vi "LHF.DB.Mongo.Util.BSONEnumToVariantArray.vi"(0 "BsonENUM":refnum<k24>, 1 "Extract _id":bool, 5 "error in (no error)":errorcluster, 8 "type":variant) -> (14 "Documents":variant[](array[variant]), 15 "ObjectIDs":string[](array[string]), 19 "error out":errorcluster)   [LabVIEW 2013, in "LHF.DB.Mongo.lvclass"]
uses:
  LHF.DB.Mongo.lvclass
  C:/Users/Ricardo/Desktop/Projetos/LabVIEW-MongoDB/src/Driver/MongoDB.Bson.dll
  Driver/MongoDB.Bson.dll
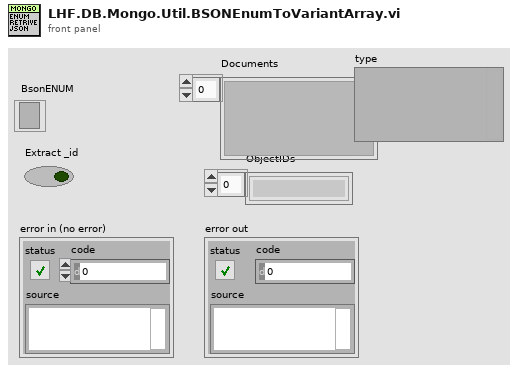
[diagram p1: front panel]
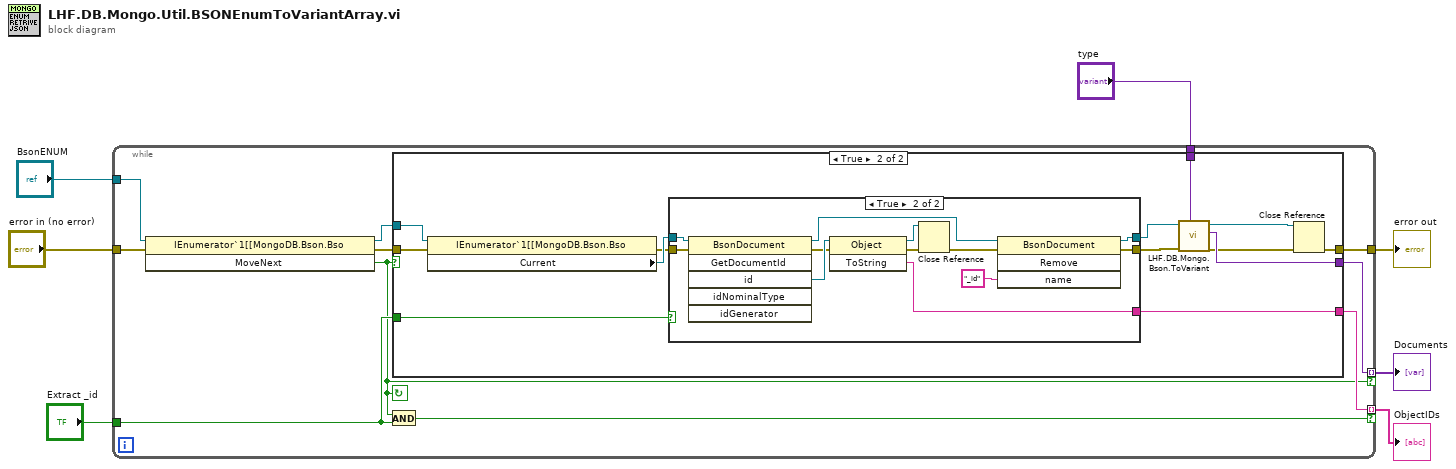
[diagram p0: block diagram]
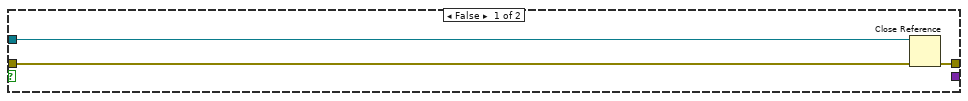
[diagram p2: hidden frame]
diagram:
  n1 = while {
    tunnel: [w16] -> w3 mode=indexing if=w10
    tunnel: [w14] -> w5
    tunnel: "error in (no error)" -> [w13]
    tunnel: "BsonENUM" -> [w18]
    tunnel: [w12] -> w6 mode=indexing if=w9
    tunnel: "Extract _id" -> [w11]
    tunnel: "type" -> [w8]
    stop <- w10 continue-if-true
    n2 = invoke class="IEnumerator`1[[MongoDB.Bson.Bso" method="MoveNext"(reference=w18, error in=w13) -> (reference out=w17:refnum<k24>, error out=w15:errorcluster, "MoveNext"=w10:bool)  [unwired: 1 in]
    n3 = And(x=w10, y=w11) -> (x .and. y?=w9:bool)
    n4 = case shown="True" w10 {
      tunnel: w17 -> [w20 w34]
      tunnel: [_ w27] -> w16
      tunnel: w15 -> [w21 w33]
      tunnel: [w19 w32] -> w14
      tunnel: [_ w31] -> w12
      tunnel: w11 -> [_ w28]
      tunnel: w8 -> [_ w26]
      frame False {
        n5 = Close Reference(reference=w20, error in (no error)=w21) -> (error out=w19:errorcluster)
      }
      frame True {
        n6 = property class="IEnumerator`1[[MongoDB.Bson.Bso"(reference=w34, error in=w33) -> (error out=w29:errorcluster, "Current"=w30:refnum<k24>)  [unwired: 1 out]
        n7 = case shown="True" w28 {
          tunnel: [_ w47] -> w31
          tunnel: w30 -> [w36 w45]
          tunnel: [w36 w44] -> w24
          tunnel: w29 -> [w35 w43]
          tunnel: [w35 w41] -> w25
          frame False {
          }
          frame True {
            n8 = invoke class="BsonDocument" method="GetDocumentId"(reference=w45, error in=w43) -> (reference out=w42:refnum<k24>, error out=w46:errorcluster, "id"=w48:refnum<k24>)  [unwired: 4 in, 3 out]
            n9 = invoke class="Object" method="ToString"(reference=w48, error in=w46) -> (reference out=w39:refnum<k24>, error out=w38:errorcluster, "ToString"=w47:string)  [unwired: 1 in]
            n10 = Close Reference(reference=w39, error in (no error)=w38) -> (error out=w37:errorcluster)
            n11 = invoke class="BsonDocument" method="Remove"(reference=w42, error in=w37, "name"="_id") -> (reference out=w44:refnum<k24>, error out=w41:errorcluster)  [unwired: 1 in, 2 out]
          }
        }
        n12 = call "LHF.DB.Mongo.Bson.ToVariant.vi"("type"=w26, "error in (no error)"=w25, "BsonValue"=w24) -> ("error out"=w22:errorcluster, "data"=w27:variant, "BsonValue 2"=w23:refnum<k24>)  [unwired: 6 in]
        n13 = Close Reference(reference=w23, error in (no error)=w22) -> (error out=w32:errorcluster)
      }
    }
  }
  "ObjectIDs" <- w6
  "error out" <- w5
  "Documents" <- w3
